vi "c_ctre_phoenix6_RequestControlMotionMagicExpoDutyCycle.vi"(0 "String 2":string, 1 "Numeric 2":u32, 2 "Numeric 3":dbl, 3 "Numeric 4":u8, 4 "Numeric 5":dbl, 5 "Numeric 6":u8, 6 "Numeric 7":dbl, 7 "Numeric 8":i32, 8 "Numeric 9":u8, 9 "Numeric 10":u8, 10 "Numeric 11":u8) -> (20 "Numeric":i32, 21 "String":string)   [LabVIEW 2023]
uses:
  <vilib>/Rock Robotics/WPI/ThirdParty/Phoenix-LabVIEW/Controls/DriverLib.ctl
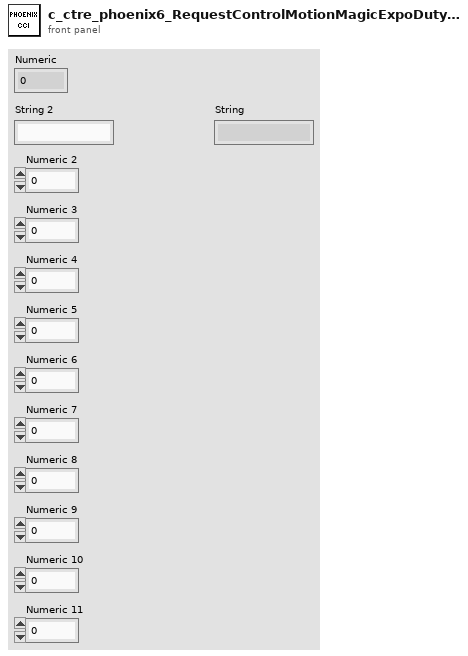
[diagram p1: front panel]
types:
  T1 = typedef "DriverLib.ctl" = path
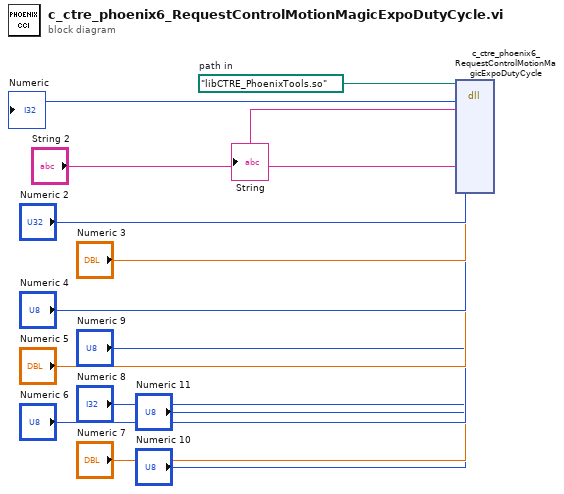
[diagram p0: block diagram]
diagram:
  w14 = T1 path "libCTRE_PhoenixTools.so"  # path in
  n1 = dll-call lib="?" fn="c_ctre_phoenix6_RequestControlMotionMagicExpoDutyCycle"(path in=w14, "String 2", "Numeric 2", "Numeric 3", "Numeric 4", "Numeric 5", "Numeric 6", "Numeric 7", "Numeric 8", "Numeric 9", "Numeric 10", "Numeric 11") -> (→"Numeric":i32, →"String":string)  [unwired: 12 in, 2 out]
